vi "MB Slave Write Input Registers (poly).vi"(1 "Starting Address":u16, 2 "Input Registers":u16[](array[numeric]), 5 "error in":errorcluster) -> (19 "error out":errorcluster)   [LabVIEW 2011]
doc: "Writes multiple input registers to the slave memory tables."
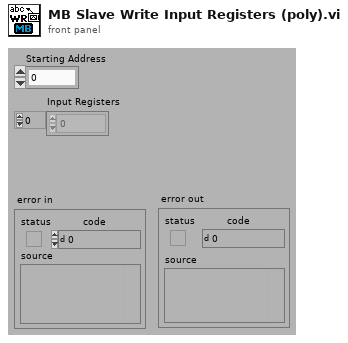
[diagram p1: front panel]
types:
  T1 = enum16{"Discrete Inputs", "Coils", "Input Registers", "Holding Registers"}
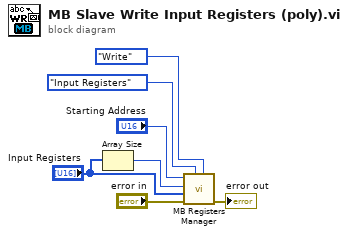
[diagram p0: block diagram]
diagram:
  n1 = Array Size(array="Input Registers") -> (size(s)=w1:i32)
  n2 = call "MB Registers Manager.vi"("Function"=enum16{"Init", "Read", "Write", "Read All"}."Write", "Table"=T1."Input Registers", "error in (no error)"="error in", "Words In"="Input Registers", "Length"=w1, "Start Address"="Starting Address") -> ("error out"=→"error out":errorcluster)  [unwired: 1 in, 4 out]
